vi "Make Snake Tail Longer.vi"(8 "error in (no error)":errorcluster, 11 "Game Board in":refnum<class "Game Board.lvclass">) -> (0 "error out":errorcluster, 3 "Game Board out":refnum<class "Game Board.lvclass">)   [LabVIEW 2018, in "Game Board.lvclass"]
uses:
  Game Board.lvclass
  Game Board.lvclass/Game Board.ctl
  Fruit/Fruit.lvclass
  Snake/Snake.lvclass
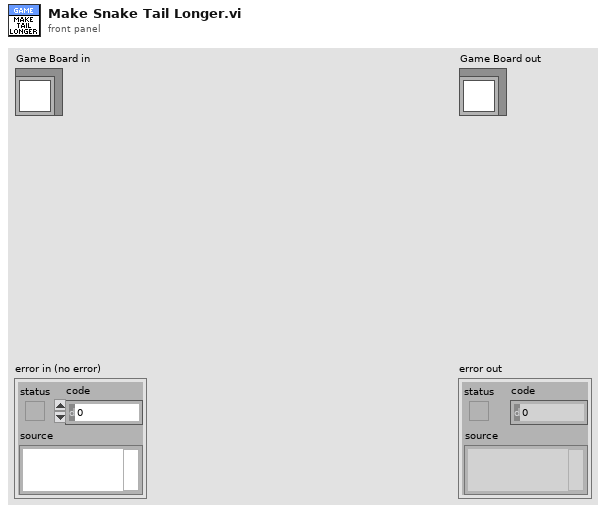
[diagram p1: front panel]
types:
  T1 = typedef "Coordinates.ctl" = cluster{"X":i32, "Y":i32}
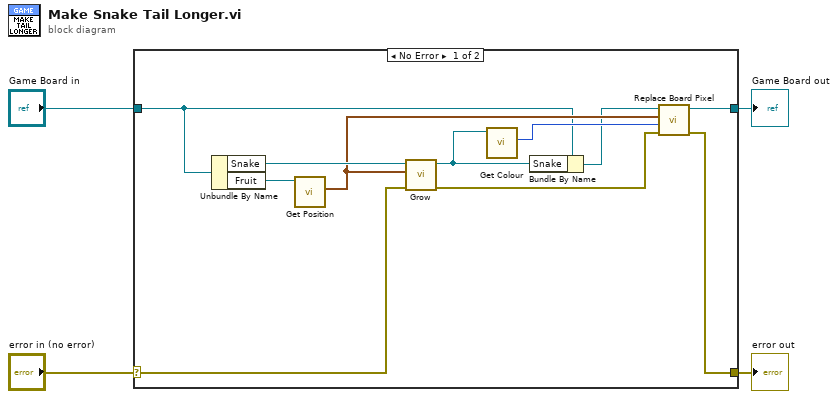
[diagram p0: block diagram]
diagram:
  n1 = case shown="No Error" "error in (no error)" {
    selector: "error in (no error)" -> [w13 w17]
    tunnel: [w5 w17] -> w3
    tunnel: [w10 w16] -> w1
    tunnel: "Game Board in" -> [w8 w16]
    frame No Error {
      n2 = Unbundle By Name(w8) -> ("Snake"=w14:refnum<class "Snake.lvclass">, "Fruit"=w15:refnum<class "Fruit.lvclass">)
      n3 = call-dynamic "Get Position.vi"("Fruit in"=w15) -> ("Coordinates"=w12:T1)  [unwired: 10 in]
      n4 = call "Grow.vi"("error in (no error)"=w13, "Coordinates"=w12, "Snake in"=w14) -> ("error out"=w6:errorcluster, "Snake out"=w7:refnum<class "Snake.lvclass">)  [unwired: 7 in]
      n5 = call-dynamic "Get Colour.vi"("Game Componants in"=w7) -> ("Componant Colour"=w11:u32)  [unwired: 10 in]
      n6 = Bundle By Name(cluster=w8, "Snake"=w7) -> (w9:refnum<class "Game Board.lvclass">)
      n7 = call "Replace Board Pixel.vi"("error in (no error)"=w6, "Colour"=w11, "Coordinates"=w12, "Game Board in"=w9) -> ("error out"=w5:errorcluster, "Game Board out"=w10:refnum<class "Game Board.lvclass">)  [unwired: 6 in]
    }
    frame Error {
    }
  }
  "error out" <- w3
  "Game Board out" <- w1
